vi "IK Benchmark.vi"() -> ()   [LabVIEW 2013, in "ikfast_labview.lvlib"]
uses:
  ikfast_labview.lvlib
  <vilib>/Analysis/baseanly.llb/Mean (DBL).vi
  <userlib>/_matio/level5/Public/Write/Append Data Element.llb/Append Data Element (1D Array of Double).vi
  <vilib>/Analysis/NI_AALBase.lvlib
  <userlib>/_matio/level5.lvlib
panel:
  in  "Data Logging":cluster{"Path":path, "Save":bool}={"Path"=path "D:/iktest.mat", "Save"=TRUE}
  out "Time (ms)":cluster{"mean":dbl, "min":dbl, "max":dbl}={"mean"=0.8783684840202332, "min"=0.0, "max"=17.013072967529297} {"max" format="%0.2f"; "min" format="%0.2f"; "mean" format="%0.2f"}
  out "Percentage":dbl=99.7787
  out "min_position":dbl[](array[numeric])=[-1.5707963267948966, -1.5707963267948966, -1.28, -1.1, -1.01, -3.141592653589793]
  out "max_position":dbl[](array[numeric])=[1.5707963267948966, 0.5235987755982988, 1.0471975511965976, 0.581, 0.675, 3.141592653589793]
  in  "ik tests":i32=1000000
  in  "Stop":bool
  out "found":i32=997787
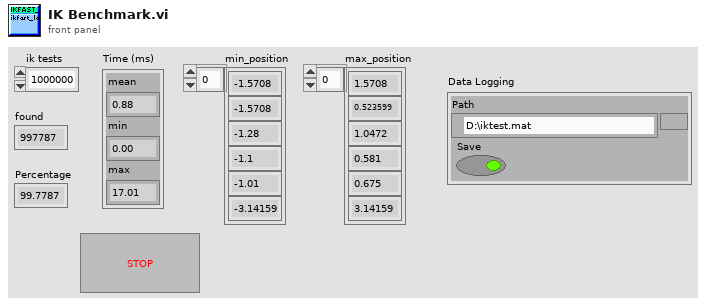
[diagram p1: front panel]
types:
  T1 = typedef "NI_Matrix.lvlib/RealMatrix.ctl" = dbl[][]
  T2 = enum16{"open", "replace", "create", "open or create", "replace or create", "replace or create with confirmation"}
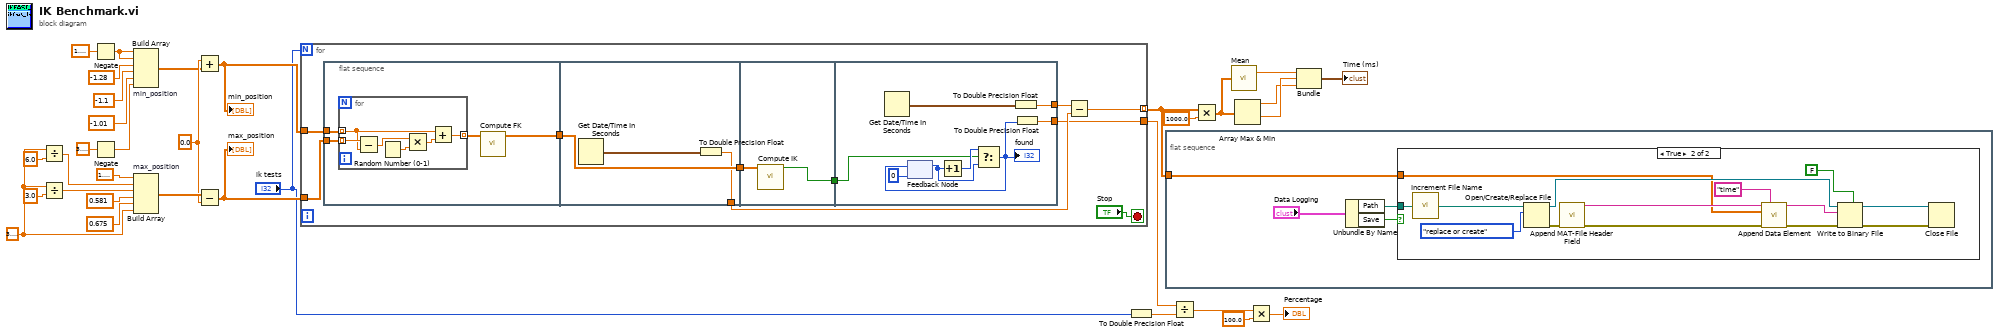
[diagram p0: block diagram]
diagram:
  w17 = 0.0 ("element")
  w19 = 3.141592653589793
  n1 = Divide(x=w19, y=6.0) -> (x/y=w24:dbl)
  n2 = Divide(x=w19, y=3.0) -> (x/y=w22:dbl)
  n3 = Negate(x=1.5707963267948966) -> (-x=w33:dbl)
  n4 = Negate(x=3.141592653589793) -> (-x=w28:dbl)
  n5 = Build Array "min_position"(w33, w33, -1.28 ("element"), -1.1 ("element"), -1.01 ("element"), w28) -> (w16:dbl[])
  n6 = Build Array "max_position"(1.5707963267948966, w24, w22, 0.581 ("element"), 0.675 ("element"), w19) -> (w18:dbl[])
  n7 = Add(x=w17, y=w16) -> (x+y=w15:dbl[])
  "min_position" <- w15
  n8 = Subtract(x=w18, y=w17) -> (x-y=w14:dbl[])
  "max_position" <- w14
  n9 = for {
    N: "ik tests" -> [_]
    tunnel: w15 -> [w43]
    tunnel: w14 -> [w42]
    tunnel: [w40] -> w2 mode=indexing
    tunnel: [w34] -> w1
    stop <- "Stop" stop-if-true
    n10 = flat-sequence {
      tunnel: w42 -> [w46]
      tunnel: w43 -> [w47]
      tunnel: [w44] -> w37
      tunnel: [w56] -> w38
      tunnel: w37 -> [w56]
      tunnel: [w54] -> w35
      tunnel: w38 -> [w58]
      tunnel: [w57] -> w36
      tunnel: [w65] -> w39
      tunnel: w36 -> [w60]
      tunnel: [w59] -> w34
      frame #0 {
        n11 = for {
          tunnel: w47 -> [w49] mode=indexing
          tunnel: w46 -> [w53] mode=indexing
          tunnel: [w48] -> w45 mode=indexing
          n12 = Subtract(x=w53, y=w49) -> (x-y=w52:dbl)
          n13 = Random Number (0-1)() -> (number: 0 to 1=w51:dbl)
          n14 = Multiply(x=w52, y=w51) -> (x*y=w50:dbl)
          n15 = Add(x=w49, y=w50) -> (x+y=w48:dbl)
        }
        n16 = call "Compute FK.vi"("joints"=w45) -> ("transform"=w44:T1)  [unwired: 9 in, 1 out]
      }
      frame #1 {
        n17 = Get Date/Time In Seconds() -> (seconds since 1Jan1904=w55:timestamp)
        n18 = To Double Precision Float(number=w55) -> (double precision float=w54:dbl)
      }
      frame #2 {
        n19 = call "Compute IK.vi"("transform"=w58) -> ("found?"=w57:bool)  [unwired: 8 in, 2 out]
      }
      frame #3 {
        n20 = Get Date/Time In Seconds() -> (seconds since 1Jan1904=w66:timestamp)
        n21 = feedback #1(0) -> (w61:i32)
        n22 = Increment(x=w61) -> (x+1=w62:i32)
        n23 = Select(t=w62, s=w60, f=w61) -> (s? t:f=w64:i32)
        "found" <- w64
        n24 = feedback-in #1(w64) -> ()
        n25 = To Double Precision Float(number=w66) -> (double precision float=w65:dbl)
        n26 = To Double Precision Float(number=w64) -> (double precision float=w59:dbl)
      }
    }
    n27 = Subtract(x=w39, y=w35) -> (x-y=w40:dbl)
  }
  n28 = To Double Precision Float(number="ik tests") -> (double precision float=w13:dbl)
  n29 = flat-sequence {
    tunnel: w2 -> [w67]
    frame #0 {
      n30 = Unbundle By Name("Data Logging") -> ("Path"=w69:path, "Save"=w68:bool)
      n31 = case shown="True" w68 {
        tunnel: w69 -> [_ w74]
        tunnel: w67 -> [_ w73]
        frame False {
        }
        frame True {
          n32 = call "Increment File Name.vi"("Full Path"=w74) -> ("New Path"=w76:path)
          n33 = Open/Create/Replace File(file path (use dialog)=w76, operation (0:open)=T2."replace or create") -> (refnum out=w77:refnum<file>, error out=w75:errorcluster)  [unwired: 4 in, 1 out]
          n34 = call <userlib>:"Append MAT-File Header Field.vi"("error"=w75) -> ("result string"=w81:string, "error out"=w80:errorcluster)  [unwired: 13 in]
          n35 = call-poly <userlib>:"Append Data Element.vi"("initial string"=w81, "Data Name"="time", "data"=w73, "error in"=w80) -> ("result string"=w72:string, "error out"=w71:errorcluster)  [unwired: 10 in]
          n36 = Write to Binary File(file (use dialog)=w77, data=w72, error in=w71, 5:FALSE ("prepend array or string size? (T)")) -> (refnum out=w83:refnum<file>, error out=w82:errorcluster)  [unwired: 2 in, 1 out]
          n37 = Close File(refnum=w83, error in=w82) -> ()  [unwired: 2 out]
        }
      }
    }
  }
  n38 = Divide(x=w1, y=w13) -> (x/y=w10:dbl)
  n39 = Multiply(x=w2, y=1000.0) -> (x*y=w7:dbl[])
  n40 = call-poly <vilib>:"Mean.vi"("X"=w7) -> ("mean"=w6:dbl)  [unwired: 1 out]
  n41 = Array Max & Min(array=w7) -> (max value=w4:dbl, min value=w5:dbl)  [unwired: 2 out]
  n42 = Multiply(x=w10, y=100.0) -> (x*y=→"Percentage":dbl)
  n43 = Bundle("mean"=w6, w5, w4) -> (→"Time (ms)":cluster{"mean":dbl, dbl, dbl})  [unwired: 1 in]
